vi "Main.vi"() -> ()   [LabVIEW 2013] (continued)
            n3896 = call <vilib>:"Application Directory.vi"() -> ("Application Directory"=w6305:path)
            n3897 = Build Path(base path=w6305, name or relative path="SRTRS.ini" ("ini Name")) -> (appended path=w6304:path)
            n3898 = call <vilib>:"Open Config Data.vi"("create file if necessary (T)"=FALSE, "configuration file path"=w6304) -> ("error out"=w6307:errorcluster, "refnum"=w6306:T59)  [unwired: 7 in, 1 out]
            n3899 = call-poly <vilib>:"Write Key.vi"("section"="Settings", "error in (no error)"=w6307, "value"="", "key"="Raw Data File", "refnum"=w6306) -> ("error out"=w6301:errorcluster, "found?"=w6300:bool, "refnum out"=w6299:T59)  [unwired: 4 in]
            n3900 = call <vilib>:"Close Config Data.vi"("error in (no error)"=w6301, "write file if changed (T)"=w6300, "refnum"=w6299) -> ("error out"=w6296:errorcluster)  [unwired: 7 in, 1 out]
            n3901 = local write "ini File Error"(w6296) -> ()
          }
        }
        n3902 = local read "Simulate cRIO"() -> (w6260:bool)
        n3903 = call "cRIO - Shared Variable RW.vi"("shared variable RT Library"=w6256, "Read/Write"=cRIO_RW_Enum."Write", "Error In"=w6258, "Simulate cRIO"=w6260, "DAQ Start"=FALSE, "cRIO Status"=w6247) -> ("Error Out"=w6261:errorcluster)  [unwired: 5 in, 8 out]
        n3904 = while {
          tunnel: w6261 -> [w6573]
          tunnel: w6260 -> [w6572]
          tunnel: w6247 -> [w6562]
          tunnel: w6256 -> [w6561]
          tunnel: [w6560] -> w6248
          i -> [w6567]
          stop <- w6569 stop-if-true
          # "Wait 5sec"
          # "Check for cRIO DAQ Stop"
          n3905 = Wait Until Next ms Multiple(millisecond multiple=u32 100) -> ()  [unwired: 1 out]
          n3906 = call "cRIO - Shared Variable RW.vi"("shared variable RT Library"=w6561, "Read/Write"=cRIO_RW_Enum."Read", "Error In"=w6573, "Simulate cRIO"=w6572, "cRIO Status"=w6562) -> ("Cycle Count"=w6570:i32, "DAQ Started"=w6563:bool, "Error Out"=w6560:errorcluster)  [unwired: 6 in, 6 out]
          n3907 = local write "cRIO Cycle Count"(w6570) -> ()
          n3908 = local write "cRIO DAQ Started"(w6563) -> ()
          n3909 = local write "cRIO Error"(w6560) -> ()
          n3910 = Not(x=w6563) -> (.not. x?=w6568:bool)
          n3911 = Greater Or Equal?(x=w6567, y=50) -> (x >= y?=w6565:bool)
          n3912 = Compound Arithmetic op=OR(w6565, w6568, w6560) -> (w6569:bool)
        }
        n3913 = global read "Global SRTRS.vi" "Logon"() -> (w6246:T21)
        n3914 = Unbundle By Name(w6246) -> ("PlantID"=w6245:string, "SystemID"=w6244:string)
        n3915 = Bundle("PlantID"=w6245, "SystemID"=w6244) -> (w6243:cluster{"PlantID":string, "SystemID":string})  [unwired: 1 in]
        n3916 = local read "DB - Transaction"() -> (w6251:bool)
        n3917 = call "Status - Update cRIO Status.vi"("Error In"=w6248, "[PlantId],[SystemId]"=w6243, "cRIO Status"=w6247) -> ("Error Out"=w6242:errorcluster)  [unwired: 8 in]
        n3918 = local write "System Status"(w6242) -> ()
        n3919 = case shown="No Error" w6249 {
          selector: w6249 -> [_ w6489]
          tunnel: w6250 -> [w6482 _]
          tunnel: [w6484 w6489] -> w6253
          frame No Error {
            # "Overwrite raw data from cRIO to Chart"
            n3920 = call "Chart - Load History.vi"("file path (dialog if empty)"=w6482) -> ("Error Out"=w6485:errorcluster, "History"=w6486:dynamicdata[])  [unwired: 5 in, 4 out]
            n3921 = property on="Chart" class="WFChart (strict)"(error in=w6485, "History Data"=w6486) -> (error out=w6484:errorcluster)  [unwired: 1 in, 1 out]
            n3922 = case shown="No Error" w6484 {
              tunnel: ["Raw Data File Load to Chart OK. " "Raw Data File Load to Chart failed. "] -> w6481
              frame No Error {
              }
              frame Error {
              }
            }
            n3923 = Path To String(path=w6482) -> (string=w6479:string)
            n3924 = Concatenate Strings("{END Recipe} ", w6481, " File: \"" ("string"), w6479, "\"" ("string")) -> (w6477:string)
            n3925 = call "Queue - EnQueue to MessageQ.vi"("<NoD> Don't Display to UI"=TRUE, "Message"=w6477) -> ()  [unwired: 9 in, 1 out]
          }
          frame Error {
          }
        }
        n3926 = case shown="True" w6251 {
          tunnel: w6250 -> [_ w6315]
          tunnel: w6249 -> [_ w6340]
          tunnel: w6241 -> [_ _]
          tunnel: w6240 -> [_ w6310]
          tunnel: [errorcluster {"status"=FALSE, "code"=0, "source"=""} ("error IO") w6314] -> w6239
          frame False {
          }
          frame True {
            w6327 = "0"  # IsActive
            w6344 = ""
            w6323 = "1"  # Process Complete
            w6360 = T62[] [enum."[EndRecordTemp]", enum."[EndRecordTime]", enum."[RecordedMinutes]", enum."[ProcessStatus]", enum."[OverallStatus]", enum."[Result]"] items=["[StartRecordTime]", "[StartRecordTemp]", "[MaxRecordedTemp]", "[MaxRecordedTempTime]", "[MinRecordedTemp]", "[MinRecordedTempTime]", "[EndRecordTemp]", "[EndRecordTime]", "[RecordedMinutes]", "[StartHoldTime]", "[StartHoldTemp]", "[HoldTimeMaxTemp]", "[HoldTimeMaxTempTime]", "[HoldTimeMinTemp]", "[HoldTimeMinTempTime]", "[EndHoldTime]", "[EndHoldTemp]", "[HoldDurationMinutes]", "[TempDiffDuringHold]", "[UnitOfTemperature]", "[PerformedBy]", "[PerformedOn]", "[IsTempWithinTol]", "[IsTimeWithinTol]", "[HoldTimePercentage]", "[ProcessStatus]", "[OverallStatus]", "[SequenceStatus]", "[Parameter1]", "[Parameter2]", "[Parameter3]", "[Parameter4]", "[Parameter5]", "[Parameter6]", "[Parameter7]", "[Parameter8]", "[Parameter9]", "[Parameter10]", "[Parameter11]", "[Parameter12]", "[Result]", "[RawDataFile]", "[RawDataFilePath]", "[RawDataFileName]", "[OutputSetId]", "[SavedBy]", "[SavedOn]", "[Inactive]"]  # [TransactionResult] Array
            # "Actuall should put whole thing in Error"
            # "Set in {Running Process} when it exited"
            n3927 = local read "[StartRecordTime]"() -> (w6355:string)
            n3928 = local read "Simulate cRIO"() -> (w6337:bool)
            n3929 = case shown="True" w6337 {
              tunnel: [w6372 w6376] -> w6336
              frame False {
                n3930 = Get Date/Time In Seconds() -> (seconds since 1Jan1904=w6372:timestamp)
              }
              frame True {
                # "Every count is 60sec"
                n3931 = local read "Process t0"() -> (w6377:timestamp)
                n3932 = local read "Samples/ch Count"() -> (w6373:i32)
                n3933 = Multiply(x=w6373, y=60) -> (x*y=w6374:i32)
                n3934 = Add(x=w6374, y=w6377) -> (x+y=w6376:timestamp)
              }
            }
            n3935 = call "Chart - Load History.vi"("file path (dialog if empty)"=w6315) -> ("t0 time stamp"=w6339:timestamp, "History"=w6338:dynamicdata[])  [unwired: 5 in, 4 out]
            n3936 = global read "Global SRTRS.vi" "Date Time Format"() -> (w6356:string)
            n3937 = call "String - Convert Str (YYYY-mm-dd HHcMMcSS) to TimeStamp.vi"("YYYY-mm-dd HH:MM:SS (String)"=w6355) -> ("time stamp"=w6335:timestamp)  [unwired: 9 in, 1 out]
            n3938 = Select(t="1", s=w6310, f="0") -> (s? t:f=w6318:string)
            n3939 = Select(t="1", s=w6310, f="0") -> (s? t:f=w6311:string)
            n3940 = Format Date/Time String(time format string (%c)=w6356, seconds (now)=w6336) -> (date/time string=w6330:string)  [unwired: 1 in]
            n3941 = local read "1st TC"() -> (w6358:dbl)
            n3942 = Subtract "Seconds"(x=w6336, y=w6335) -> (x-y=w6354:dbl)
            n3943 = Divide "Minutes"(x=w6354, y=60.0) -> (x/y=w6352:dbl)
            n3944 = Format Value(format string="%#_4", value (0)=w6358) -> (output string=w6357:string)  [unwired: 1 in]
            n3945 = Number To Decimal String(number=w6352) -> (decimal integer string=w6329:string)  [unwired: 1 in]
            n3946 = Build Array(w6357, w6330, w6329, w6323, w6318, w6311) -> (w6351:string[])
            n3947 = control-ref of="Process Completed"() -> (w6322:refnum<vi>)
            n3948 = control-ref of="Overall Status"() -> (w6317:refnum<vi>)
            n3949 = call "String - Boolean Ref Color.vi"("Bool Refnum"=w6322) -> ("Color (U32 String)"=w6321:string)  [unwired: 4 in]
            n3950 = call "String - Boolean Ref Color.vi"("Bool Refnum"=w6317) -> ("Color (U32 String)"=w6316:string)  [unwired: 4 in]
            n3951 = local read "Transaction No (Execute)"() -> (w6342:string)
            n3952 = local read "TransactionRunNo (Execute)"() -> (w6341:string)
            n3953 = Build Array(w6330, w6329, w6321, w6316, w6327) -> (w6328:string[])
            n3954 = Bundle("Transaction No (Execute)"=w6342, "TransactionRunNo (Execute)"=w6341) -> (w6334:T77)  [unwired: 1 in]
            n3955 = global read "Global SRTRS.vi" "Logon"() -> (w6346:T21)
            n3956 = call "DB - [Execute].[Transaction].vi"("DB.Schema.Table"="SRTRS.Execute.TransactionResult", "Transaction"=w6334, "DB - Execute Transaction"=DB_-_Execute_Transaction_Enum."UPDATE [TransactionResult]", "[TransactionResult] v02"=w6360, "<Values>"=w6351) -> ("SUMMARY"=w6347:errorcluster)  [unwired: 11 in, 3 out]
            n3957 = Unbundle By Name(w6346) -> ("PlantID"=w6349:string, "StationID"=w6348:string)
            n3958 = Build Array(w6349, w6348, w6344, w6344) -> (w6345:string[])
            n3959 = local read "Enable Central Monitoring"() -> (w6332:bool)
            n3960 = local read "DB - Active Process"() -> (w6333:bool)
            n3961 = call "DB - [Execute].[Transaction].vi"("DB.Schema.Table"="SRTRS.Execute.Active", "error in (no error)"=w6347, "DB - Execute Transaction"=DB_-_Execute_Transaction_Enum."INSERT/UPDATE [Execute].[Active]", "<Values>"=w6345) -> ("SUMMARY"=w6326:errorcluster)  [unwired: 12 in, 3 out]
            n3962 = And(x=w6332, y=w6333) -> (x .and. y?=w6331:bool)
            n3963 = case shown="True" w6331 {
              tunnel: w6328 -> [_ w6367]
              tunnel: [_ w6366] -> w6324
              frame False {
              }
              frame True {
                w6371 = T63[] [enum."[EndRecordTime]", enum."[RecordedMinutes]", enum."[ProcessColor]", enum."[OverallColor]", enum."[IsActive]"] items=["[IsActive]", "[TransactionNo]", "[TransactionRunNo]", "[SequenceStatus]", "[StartRecordTime]", "[EndRecordTime]", "[StartHoldTime]", "[EndHoldTime]", "[Message1]", "[Message2]", "[HoldTimeRemaining]", "[HoldTimePercentage]", "[HoldProgressColor]", "[OrderNumbers]", "[CurrentTemp]", "[UnitOfTemperature]", "[IsAppClientLive]", "[RawDataFile]", "[RecordedMinutes]", "[FurnaceControlStatus]", "[FurnaceControlColor]", "[ControllerStatus]", "[ControllerColor]", "[IsControllerOnline]", "[ProcessColor]", "[OverallColor]", "[LastUpdatedOn]", "[LastUpdatedCmsTime]", "[Inactive]"] ("[Execute].[ActiveProcess]\n2014-10-14 14:58")
                n3964 = global read "Global SRTRS.vi" "Logon"() -> (w6370:T21)
                n3965 = Unbundle By Name(w6370) -> ("PlantID"=w6369:string, "SystemID"=w6368:string)
                n3966 = Bundle("PlantID"=w6369, "SystemID"=w6368) -> (w6365:cluster{"PlantID":string, "SystemID":string})  [unwired: 1 in]
                n3967 = call "DB - [CMS].[Execute].[ActiveProcess].vi"("Application"="SRTRS", "[PlantId],[SystemId]"=w6365, "DB - CMS Execute ActiveProcess"=DB_-_CMS_Execute_Active_Process."UPDATE [Execute].[ActiveProcess]", "[Execute].[ActiveProcess]\n2014-10-14 14:58"=w6371, "<Data>"=w6367) -> ("SUMMARY"=w6366:errorcluster)  [unwired: 11 in, 3 out]
              }
            }
            n3968 = Merge Errors(w6324, w6326) -> (w6325:errorcluster)
            n3969 = case shown="No Error" w6340 {
              selector: w6340 -> [_ w6475]
              tunnel: w6338 -> [w6471 _]
              tunnel: w6339 -> [w6465 _]
              tunnel: w6325 -> [_ _]
              tunnel: w6334 -> [w6442 _]
              tunnel: w6315 -> [w6409 _]
              tunnel: [w6399 w6475] -> w6314
              frame No Error {
                w6440 = "%#_4" ("format string")
                w6423 = T62[] [enum."[MaxRecordedTemp]", enum."[MaxRecordedTempTime]", enum."[MinRecordedTemp]", enum."[MinRecordedTempTime]", enum."[TempDiffDuringHold]"] items=["[StartRecordTime]", "[StartRecordTemp]", "[MaxRecordedTemp]", "[MaxRecordedTempTime]", "[MinRecordedTemp]", "[MinRecordedTempTime]", "[EndRecordTemp]", "[EndRecordTime]", "[RecordedMinutes]", "[StartHoldTime]", "[StartHoldTemp]", "[HoldTimeMaxTemp]", "[HoldTimeMaxTempTime]", "[HoldTimeMinTemp]", "[HoldTimeMinTempTime]", "[EndHoldTime]", "[EndHoldTemp]", "[HoldDurationMinutes]", "[TempDiffDuringHold]", "[UnitOfTemperature]", "[PerformedBy]", "[PerformedOn]", "[IsTempWithinTol]", "[IsTimeWithinTol]", "[HoldTimePercentage]", "[ProcessStatus]", "[OverallStatus]", "[SequenceStatus]", "[Parameter1]", "[Parameter2]", "[Parameter3]", "[Parameter4]", "[Parameter5]", "[Parameter6]", "[Parameter7]", "[Parameter8]", "[Parameter9]", "[Parameter10]", "[Parameter11]", "[Parameter12]", "[Result]", "[RawDataFile]", "[RawDataFilePath]", "[RawDataFileName]", "[OutputSetId]", "[SavedBy]", "[SavedOn]", "[Inactive]"] ("[TransactionResult] v02")
                w6443 = "%#_4" ("format string")
                w6424 = T62[] [enum."[HoldTimeMaxTemp]", enum."[HoldTimeMaxTempTime]", enum."[HoldTimeMinTemp]", enum."[HoldTimeMinTempTime]", enum."[TempDiffDuringHold]"] items=["[StartRecordTime]", "[StartRecordTemp]", "[MaxRecordedTemp]", "[MaxRecordedTempTime]", "[MinRecordedTemp]", "[MinRecordedTempTime]", "[EndRecordTemp]", "[EndRecordTime]", "[RecordedMinutes]", "[StartHoldTime]", "[StartHoldTemp]", "[HoldTimeMaxTemp]", "[HoldTimeMaxTempTime]", "[HoldTimeMinTemp]", "[HoldTimeMinTempTime]", "[EndHoldTime]", "[EndHoldTemp]", "[HoldDurationMinutes]", "[TempDiffDuringHold]", "[UnitOfTemperature]", "[PerformedBy]", "[PerformedOn]", "[IsTempWithinTol]", "[IsTimeWithinTol]", "[HoldTimePercentage]", "[ProcessStatus]", "[OverallStatus]", "[SequenceStatus]", "[Parameter1]", "[Parameter2]", "[Parameter3]", "[Parameter4]", "[Parameter5]", "[Parameter6]", "[Parameter7]", "[Parameter8]", "[Parameter9]", "[Parameter10]", "[Parameter11]", "[Parameter12]", "[Result]", "[RawDataFile]", "[RawDataFilePath]", "[RawDataFileName]", "[OutputSetId]", "[SavedBy]", "[SavedOn]", "[Inactive]"] ("[TransactionResult] v02")
                w6468 = u16 1 items=["Samples", "Relative Time"] ("start/duration format")
                w6469 = 0  # TC0
                # "Use this Sequence with Recovery Flag to update \n- Variant Hold Time (Indicator)\n- Varaint Hold Temp (Indicator)\n- Overall Status (Indicator)\n- OverallStatus & Result (DB)\n(Already computed - ProcessStatus (DB))"
                # "Calculate Parameters from FTP-ed raw data from cRIO"
                n3970 = local read "Parameter Buffer"() -> (w6474:T15)
                n3971 = Unbundle By Name(w6474) -> ("Start Holding Time and Date"=w6473:string, "End Holding Time and Date"=w6472:string)  [unwired: 2 out]
                n3972 = Index Array(array=w6471, index=w6469) -> (element=w6470:dynamicdata)
                n3973 = call "Convert from Dynamic Data"("Dynamic Data Type"=w6470) -> ("Waveform"=w6441:waveform(dbl))  [unwired: 3 in]
                n3974 = call "String - Convert Str (YYYY-mm-dd HHcMMcSS) to TimeStamp.vi"("YYYY-mm-dd HH:MM:SS (String)"=w6473) -> ("time stamp"=w6467:timestamp)  [unwired: 9 in, 1 out]
                n3975 = call "String - Convert Str (YYYY-mm-dd HHcMMcSS) to TimeStamp.vi"("YYYY-mm-dd HH:MM:SS (String)"=w6472) -> ("time stamp"=w6466:timestamp)  [unwired: 9 in, 1 out]
                n3976 = Subtract(x=w6467, y=w6465) -> (x-y=w6463:dbl)
                n3977 = Subtract(x=w6466, y=w6465) -> (x-y=w6464:dbl)
                n3978 = Subtract(x=w6464, y=w6463) -> (x-y=w6397:dbl)
                n3979 = call-poly <vilib>:"Get Waveform Subset.vi"("start/duration format"=w6468, "duration"=w6397, "start samples/time"=w6463, "waveform in"=w6441) -> ("error out"=→"Chart":errorcluster, "waveform out"=w6461:waveform(dbl))  [unwired: 2 in, 2 out]
                n3980 = Divide "Hold Time (min)"(x=w6397, y=60.0) -> (x/y=w6395:dbl)
                n3981 = call "Statistics"("Signals"=w6461) -> ("Range"=w6455:dynamicdata, "Time of Minimum"=w6456:dynamicdata, "Minimum"=w6457:dynamicdata, "Time of Maximum"=w6458:dynamicdata, "Maximum"=w6459:dynamicdata, "error out"=w6417:errorcluster)  [unwired: 21 in]
                n3982 = call "Statistics2"("Signals"=w6441) -> ("Time of Minimum"=w6429:dynamicdata, "Minimum"=w6430:dynamicdata, "Time of Maximum"=w6431:dynamicdata, "Maximum"=w6432:dynamicdata, "error out"=w6416:errorcluster)  [unwired: 21 in, 1 out]
                n3983 = property on="Variant Allowed (Hold Temp)" class="DigNum (strict)"() -> ("Value"=w6380:dbl)  [unwired: 2 in, 2 out]
                n3984 = property on="Hold. Temp." class="Str"() -> ("Value"=w6390:string)  [unwired: 2 in, 2 out]
                n3985 = property on="Variant Allowed (Hold Time)" class="DigNum (strict)"() -> ("Value"=w6392:dbl)  [unwired: 2 in, 2 out]
                n3986 = property on="Hold. Time (hour:minute)" class="Str"() -> ("Value"=w6398:string)  [unwired: 2 in, 2 out]
                n3987 = Merge Errors(w6417, w6416) -> (→"Statistics":errorcluster)
                n3988 = call "String - (HH_colon_MM) to Minutes.vi"("Hold Time (HH:MM)"=w6398) -> ("minutes"=w6394:dbl)  [unwired: 10 in]
                n3989 = call "Convert from Dynamic Data7"("Dynamic Data Type"=w6432) -> ("Scalar"=w6428:dbl)  [unwired: 3 in]
                n3990 = call "Convert from Dynamic Data8"("Dynamic Data Type"=w6431) -> ("Scalar"=w6427:dbl)  [unwired: 3 in]
                n3991 = call "Convert from Dynamic Data9"("Dynamic Data Type"=w6430) -> ("Scalar"=w6426:dbl)  [unwired: 3 in]
                n3992 = call "Convert from Dynamic Data10"("Dynamic Data Type"=w6429) -> ("Scalar"=w6425:dbl)  [unwired: 3 in]
                n3993 = call "Convert from Dynamic Data2"("Dynamic Data Type"=w6459) -> ("Scalar"=w6389:dbl)  [unwired: 3 in]
                n3994 = call "Convert from Dynamic Data3"("Dynamic Data Type"=w6458) -> ("Scalar"=w6453:dbl)  [unwired: 3 in]
                n3995 = call "Convert from Dynamic Data4"("Dynamic Data Type"=w6457) -> ("Scalar"=w6388:dbl)  [unwired: 3 in]
                n3996 = call "Convert from Dynamic Data5"("Dynamic Data Type"=w6456) -> ("Scalar"=w6454:dbl)  [unwired: 3 in]
                n3997 = call "Convert from Dynamic Data6"("Dynamic Data Type"=w6455) -> ("Scalar"=w6445:dbl)  [unwired: 3 in]
                n3998 = global read "Global SRTRS.vi" "Date Time Format"() -> (w6433:string)
                n3999 = Fract/Exp String To Number(string=w6390) -> (number=w6387:dbl)  [unwired: 3 in, 1 out]
                n4000 = To Time Stamp(1:w6427) -> (0:w6434:timestamp)
                n4001 = To Time Stamp(1:w6453) -> (0:w6452:timestamp)
                n4002 = To Time Stamp(1:w6425) -> (0:w6436:timestamp)
                n4003 = To Time Stamp(1:w6454) -> (0:w6450:timestamp)
                n4004 = Subtract(x=w6395, y=w6394) -> (x-y=w6393:dbl)
                n4005 = Absolute Value(x=w6393) -> (abs(x)=w6391:dbl)
                "|Hold - Hold Time|" <- w6391
                n4006 = Format Value(format string=w6440, value (0)=w6428) -> (output string=w6438:string)  [unwired: 1 in]
                n4007 = Format Date/Time String(time format string (%c)=w6433, seconds (now)=w6434) -> (date/time string=w6435:string)  [unwired: 1 in]
                n4008 = Format Value(format string=w6443, value (0)=w6389) -> (output string=w6447:string)  [unwired: 1 in]
                n4009 = Format Date/Time String(time format string (%c)=w6433, seconds (now)=w6452) -> (date/time string=w6451:string)  [unwired: 1 in]
                n4010 = Format Value(format string=w6440, value (0)=w6426) -> (output string=w6439:string)  [unwired: 1 in]
                n4011 = Format Date/Time String(time format string (%c)=w6433, seconds (now)=w6436) -> (date/time string=w6437:string)  [unwired: 1 in]
                n4012 = Format Value(format string=w6443, value (0)=w6388) -> (output string=w6446:string)  [unwired: 1 in]
                n4013 = Format Date/Time String(time format string (%c)=w6433, seconds (now)=w6450) -> (date/time string=w6449:string)  [unwired: 1 in]
                n4014 = Format Value(format string=w6443, value (0)=w6445) -> (output string=w6444:string)  [unwired: 1 in]
                n4015 = Greater?(x=w6392, y=w6391) -> (0:→"Variant Allowed (Hold Time) (raw Data)":bool)
                n4016 = Build Array(w6438, w6435, w6439, w6437) -> (w6421:string[])
                n4017 = Build Array(w6447, w6451, w6446, w6449, w6444) -> (w6420:string[])
                n4018 = Build Array (concatenate)(w6420, w6421) -> (w6419:string[])
                "Calculate Parameters from raw Data" <- w6419
                n4019 = Subtract(x=w6389, y=w6387) -> (x-y=w6386:dbl)
                n4020 = Subtract(x=w6388, y=w6387) -> (x-y=w6385:dbl)
                n4021 = Absolute Value(x=w6386) -> (abs(x)=w6378:dbl)
                "|Max - Hold Temp|" <- w6378
                n4022 = Absolute Value(x=w6385) -> (abs(x)=w6379:dbl)
                "|Min - Hold Temp|" <- w6379
                n4023 = Greater?(x=w6380, y=w6378) -> (0:w6384:bool)
                n4024 = Greater?(x=w6380, y=w6379) -> (0:w6383:bool)
                n4025 = And(x=w6384, y=w6383) -> (x .and. y?=→"Variant Allowed (Hold Temp) (raw Data)":bool)
                n4026 = Build Array (concatenate)(w6424, w6423) -> (w6422:T62[])
                n4027 = call "DB - [Execute].[Transaction].vi"("DB.Schema.Table"="SRTRS.Execute.TransactionResult", "Transaction"=w6442, "DB - Execute Transaction"=DB_-_Execute_Transaction_Enum."UPDATE [TransactionResult]", "[TransactionResult] v02"=w6422, "<Values>"=w6419) -> ("Transaction"=w6402:T19, "SUMMARY"=w6404:errorcluster)  [unwired: 11 in, 2 out]
                n4028 = Open/Create/Replace File(file path (use dialog)=w6409, access (0:read/write)=enum16{"read/write", "read-only", "write-only"}."read-only") -> (refnum out=w6408:refnum<file>)  [unwired: 4 in, 2 out]
                n4029 = Set File Position(refnum=w6408, from (0:start)=enum16{"start", "end", "current"}."start") -> (refnum out=w6412:refnum<file>, error out=w6413:errorcluster)  [unwired: 2 in]
                n4030 = Read from Text File(file (use dialog)=w6412, count=-1, error in=w6413) -> (refnum out=w6405:refnum<file>, text=w6407:string, error out=w6406:errorcluster)  [unwired: 1 in, 1 out]
                n4031 = call "DB - [Execute].[Transaction].vi"("DB.Schema.Table"="SRTRS.Execute.TransactionResult", "String ([RawDataFile] Filestream)"=w6407, "Transaction"=w6402, "error in (no error)"=w6404, "DB - Execute Transaction"=DB_-_Execute_Transaction_Enum."UPDATE FILESTREAM") -> ("SUMMARY"=w6401:errorcluster)  [unwired: 11 in, 3 out]
                n4032 = local write "DB"(w6401) -> ()
                n4033 = Close File(refnum=w6405, error in=w6406) -> (error out=w6400:errorcluster)  [unwired: 1 out]
                n4034 = local write "Data File Error"(w6400) -> ()
                n4035 = Merge Errors(w6401, w6400) -> (w6399:errorcluster)
              }
              frame Error {
              }
            }
          }
        }
        n4036 = case shown="True" "Report.Create.Excel" {
          tunnel: w6259 -> [w6574 _]
          tunnel: [w6574 w6575] -> w6265
          tunnel: w6250 -> [_ w6576]
          tunnel: w6239 -> [_ _]
          frame False {
          }
          frame True {
            # "Create Excel Report"
            n4037 = flat-sequence {
              tunnel: w6576 -> [w6581]
              tunnel: [w6582] -> w6575
              frame #0 {
                # "Update Correct Transaction for Report\nSince this is immediately after a \nRUN, we will use the (Execute's) \nTranscation"
                # "This the raw data file from cRIO\n(unless cRIO is simulated)"
                n4038 = local write "Raw Data File (Report Tab)"(w6581) -> ()
                n4039 = local read "TransactionRunNo (Execute)"() -> (w6579:string)
                n4040 = local read "Transaction No (Execute)"() -> (w6580:string)
                n4041 = global read "Global SRTRS.vi" "Logon"() -> (→"Logon (Report Buffer)":T21)
                n4042 = Bundle("Transaction No (Execute)"=w6580, "TransactionRunNo (Execute)"=w6579) -> (→"Transaction (Report Buffer)":T77)  [unwired: 1 in]
              }
              frame #1 {
                # "Check if Dwell completed.\nIf not, most likely, user pressed\nStop Button"
                n4043 = local read "Parameter (End Dwell Time)"() -> (w6583:timestamp)
                n4044 = Equal?(x=w6583, y=timestamp(3471350400 s since 1904-01-01) ("Parameter (Start Dwell Time)")) -> (x = y?=w6585:bool)
                n4045 = case shown="False" w6585 {
                  tunnel: [TRUE ("T button?") w6600] -> w6586
                  frame False {
                    # "Hold Complete"
                  }
                  frame True {
                    # "Prompt for Report Generation if Hold NOT Complete"
                    n4046 = call "Msgbox - Message Handler.vi"("Short Description (When DB Not Available)"="Generate Report?", "Description (When DB Not Available)"="Hold process did not complete. Do you want to generate report?", "<.?....> Message Code"="<W 308>") -> ("MHandler Error"=w6601:errorcluster, "OK Out"=w6600:bool)  [unwired: 6 in, 1 out]
                    n4047 = local write "MHandler"(w6601) -> ()
                  }
                }
                n4048 = case shown="True" w6586 {
                  tunnel: [errorcluster {"status"=FALSE, "code"=0, "source"=""} ("error out") w6593] -> w6582
                  frame False {
                    n4049 = call "Queue - EnQueue to MessageQ.vi"("<NoD> Don't Display to UI"=TRUE, "Message"="{END Recipe} Generate Report. User click Cancel.") -> ()  [unwired: 9 in, 1 out]
                  }
                  frame True {
                    n4050 = local read "ReportList Cluster"() -> (w6592:T18)
                    n4051 = Bundle By Name(cluster=w6592, "[IsManual]"="0") -> (w6591:T18)
                    n4052 = local write "ReportList Cluster"(w6591) -> ()
                    n4053 = property on="Report Generate Toggle" class="Bool (strict)"() -> ("Value"=w6594:bool)  [unwired: 2 in, 2 out]
                    n4054 = Not(x=w6594) -> (.not. x?=w6595:bool)
                    n4055 = property on="Report Generate Toggle" class="Bool (strict)"("Val(Sgnl)"=w6595) -> (error out=w6593:errorcluster)  [unwired: 2 in, 1 out]
                  }
                }
              }
            }
          }
        }
        n4056 = Merge Errors(w6265) -> (w6264:errorcluster)
      }
      frame "ERROR Handling" {
        # "Segment.Type"
        # "Wait For RUN"
        # "State. Must always connect"
        # "Cycle Count. Not in use but leave it for future"
        # "Must Keep Sample/ch Count because the Error may have \ncome from RUNNING Process 1. We need to keep track\non the Count."
        # "Clear Error \nUnless MessageQ has an Error\nin which case the Program \nWill Quit"
        # "Clear Error, STOP Processes"
        n4057 = Unbundle By Name(w6606) -> ("code"=w6609:i32)
        n4058 = flat-sequence {
          frame #0 {
            # "STOP cRIO"
          }
        }
        n4059 = case shown="0, Default" w6609 {
          tunnel: [w6618 _] -> w6608
          tunnel: [_ w6673] -> w6607
          tunnel: [_ w6672] -> _
          tunnel: w6606 -> [w6613 _]
          tunnel: w6605 -> [w6620 _]
          frame 0, Default {
            # "Error From ET3500 and cRIO"
            # "State with Error"
            # "-1950679035"
            # "-1073807193"
            # "Normal Error, \nNot Serious, we clear error and go back to READY TO START"
            n4060 = local read "Show LabVIEW Error"() -> (w6621:bool)
            n4061 = local read "ET3500 Error"() -> (w6614:errorcluster)
            n4062 = local read "Data File Error"() -> (w6611:errorcluster)
            n4063 = local read "cRIO Error"() -> (w6615:errorcluster)
            n4064 = Merge Errors(w6615, w6614) -> (w6623:errorcluster)
            n4065 = disable-structure shown="Disabled" {
              frame Disabled {
                w6653 = T35 [enum."Page Enabled", enum."Page Enabled", enum."Page Enabled", enum."Page Enabled", enum."Page Enabled"] items=["Page Enabled", "Page Disabled", "Page Disabled & Grayed"]
                n4066 = property on="Tab Body" class="TabCtl (strict)"() -> ("Pages"=w6654:refnum<vi>[])  [unwired: 2 in, 2 out]
                n4067 = for {
                  tunnel: w6654 -> [w6656] mode=indexing
                  tunnel: w6653 -> [w6655] mode=indexing
                  n4068 = property class="Page"(reference=w6656, "PageEnb"=w6655) -> ()  [unwired: 1 in, 2 out]
                }
              }
              frame Enabled {
              }
            }
            n4069 = case shown="False" w6621 {
              tunnel: w6613 -> [_ w6652]
              frame False {
              }
              frame True {
                n4070 = call <vilib>:"Simple Error Handler.vi"("error in (no error)"=w6652) -> ()  [unwired: 4 in, 5 out]
              }
            }
            n4071 = case shown="Error" w6611 {
              selector: w6611 -> [_ w6627]
              tunnel: [_ w6624] -> w6610
              frame No Error {
              }
              frame Error {
                n4072 = Unbundle By Name(w6627) -> ("source"=w6625:string)  [unwired: 1 out]
                n4073 = Concatenate Strings(" File I/O  ERROR. \n" ("element"), w6625) -> (w6624:string)
              }
            }
            n4074 = case shown="Error" w6614 {
              selector: w6614 -> [_ w6671]
              tunnel: [_ w6668] -> w6617
              frame No Error {
              }
              frame Error {
                n4075 = Unbundle By Name(w6671) -> ("source"=w6669:string)  [unwired: 1 out]
                n4076 = control-ref of="ET3504 Status"() -> (w6666:refnum<vi>)
                n4077 = property class="Str"(reference=w6666, "Text.BG Color"=u32 16777216 ("ET3500 Transparent Color"), "Value"="Offline." ("ET3500 Program Status")) -> ()  [unwired: 1 in, 2 out]
                n4078 = Concatenate Strings(" ET3500 comm ERROR. \n" ("element"), w6669, "\n\n" ("string")) -> (w6668:string)
              }
            }
            n4079 = case shown="Error" w6615 {
              selector: w6615 -> [_ w6663]
              tunnel: [_ w6660] -> w6616
              frame No Error {
              }
              frame Error {
                n4080 = Unbundle By Name(w6663) -> ("source"=w6661:string)  [unwired: 1 out]
                n4081 = control-ref of="cRIO Status"() -> (w6658:refnum<vi>)
                n4082 = property class="Str"(reference=w6658, "Text.BG Color"=u32 16777216 ("ET3500 Transparent Color"), "Value"="Offline. " ("cRIO Status")) -> ()  [unwired: 1 in, 2 out]
                n4083 = Concatenate Strings(" cRIO comm ERROR. \n" ("element"), w6661) -> (w6660:string)
              }
            }
            n4084 = Unbundle By Name(w6613) -> ("source"=w6612:string)
            n4085 = Concatenate Strings(w6610, w6616, w6617) -> (w6622:string)
            n4086 = case shown="\"READY TO START\", Default" w6620 {
              tunnel: w6623 -> [w6632 w6642]
              tunnel: w6622 -> [w6631 w6644]
              tunnel: [errorcluster {"status"=FALSE, "code"=0, "source"=""} ("ET3500 Error") _] -> w6619
              tunnel: [Enum_-_SRTRS_State."READY TO START" ("Enum") Enum_-_SRTRS_State."RUNNING Process" ("Enum")] -> w6618
              tunnel: w6612 -> [_ w6643]
              frame "READY TO START", Default {
                # "Prompt Error"
                n4087 = case shown="Error" w6632 {
                  tunnel: w6631 -> [_ w6640]
                  frame No Error {
                  }
                  frame Error {
                    # "Error for cRIO and ET3500 ONLY\nFile I/O Error logged in their respective State."
                    n4088 = Concatenate Strings("{Error Handling}" ("string"), w6640) -> (w6634:string)
                    n4089 = local write "Tab Body"(Enum_-_Tabs."Setup" ("Tab Body")) -> ()
                    n4090 = call "Msgbox - Message Handler.vi"("Short Description (When DB Not Available)"="Communication Error", "Description (When DB Not Available)"="Cannot start process.", "<.?....> Message Code"="<E 301>") -> ("MHandler Error"=w6635:errorcluster)  [unwired: 6 in, 2 out]
                    n4091 = local write "MHandler"(w6635) -> ()
                    n4092 = call "Queue - EnQueue to MessageQ.vi"("<NoD> Don't Display to UI"=TRUE, "Message"=w6634) -> ()  [unwired: 9 in, 1 out]
                  }
                }
              }
              frame "RUNNING Process" {
                # "Continue to go back to the same STATE. \nOnly Status will update that there is an ERROR. User can still choose to STOP the Recipe or CLOSE the program."
                n4093 = case shown="Error" w6642 {
                  tunnel: w6644 -> [_ w6650]
                  tunnel: w6643 -> [_ w6648]
                  frame No Error {
                  }
                  frame Error {
                    # "For cRIO (and ET3500) Errors Only\nFile I/O error Logged at respective States"
                    n4094 = Concatenate Strings("{Error Handling} " ("element"), w6650, " {Error Source} " ("string"), w6648) -> (w6647:string)
                    n4095 = call "Queue - EnQueue to MessageQ.vi"("<NoD> Don't Display to UI"=TRUE, "Message"=w6647) -> ()  [unwired: 9 in, 1 out]
                  }
                }
              }
            }
            n4096 = flat-sequence {
              tunnel: w6619 -> [w6628]
              frame #0 {
                n4097 = local write "ET3500 Error"(w6628) -> ()
                n4098 = local write "Data File Error"(w6628) -> ()
                n4099 = local write "cRIO Error"(w6628) -> ()
              }
            }
          }
          frame -88888 {
            w6672 = " QUIT."  # Send to MessageQ
            w6673 = TRUE  # STOP While Loop
            # "No more next STATE"
            # "Serious Error,  QUIT Now"
          }
        }
        n4100 = flat-sequence {
          frame #0 {
            # "Clear RS232"
          }
        }
      }
      frame "QUIT" {
        # "IS THIS TRUE OR FALSE?"
        # "Nothing to STOP at ET3500 because the only iteraction is via cRIO COM port which\nis controlled by the HOST. Once the HOST stops, no more COM commands will be issued."
        # "Clear All Hardware States"
        n4101 = flat-sequence {
          frame #0 {
            n4102 = local read "cRIO DAQ Started"() -> (w6676:bool)
            n4103 = case shown="True" w6676 {
              frame False {
              }
              frame True {
                # "Stop DAQ Start"
                # "If cRIO DAQ Started already"
                n4104 = local read "cRIO shared variable RT Library"() -> (w6678:string)
                n4105 = local read "Simulate cRIO"() -> (w6681:bool)
                n4106 = control-ref of="cRIO Status"() -> (w6679:refnum<vi>)
                n4107 = call "cRIO - Shared Variable RW.vi"("shared variable RT Library"=w6678, "Read/Write"=cRIO_RW_Enum."Write", "Simulate cRIO"=w6681, "DAQ Start"=FALSE, "cRIO Status"=w6679) -> ("Error Out"=w6680:errorcluster)  [unwired: 6 in, 8 out]
                n4108 = local write "cRIO Error"(w6680) -> ()
              }
            }
            n4109 = local write "Quit Flag"(TRUE ("Quit Flag")) -> ()
          }
          frame #1 {
            n4110 = call "Queue - EnQueue to MessageQ.vi"("<NoD> Don't Display to UI"=TRUE, "Message"="QUIT" ("element")) -> ()  [unwired: 9 in, 1 out]
          }
        }
      }
    }
    "State Machine Error Out" <- w4367
    n4111 = Format Date/Time String(time format string (%c)="%b %d, %Y  %H:%M:%S") -> (date/time string=→"date/time string":string)  [unwired: 2 in]
    n4112 = case shown="No Error" w4367 {
      tunnel: w4371 -> [w4380 _]
      tunnel: [w4375 Enum_-_SRTRS_State."ERROR Handling" ("Enum")] -> w4366
      frame No Error {
        n4113 = local read "Recipe Stop Flag"() -> (w4374:bool)
        n4114 = local read "Quit Flag"() -> (w4373:bool)
        n4115 = Or(x=w4374, y=w4373) -> (x .or. y?=w4379:bool)
        n4116 = Select(t=Enum_-_SRTRS_State."END Recipe" ("Enum"), s=w4374, f=Enum_-_SRTRS_State."QUIT" ("Enum")) -> (s? t:f=w4376:T22)
        n4117 = Select(t=w4376, s=w4379, f=w4380) -> (s? t:f=w4375:T22)
      }
      frame Error {
      }
    }
    "StateMachine for Main Process" <- w4363
  }
  n4118 = disable-structure "Templates" shown="Disabled" {
    frame Disabled {
      w6689 = "{Save WPS Cancelled} ... must be entered." ("element")
      (unwired) path "C:/Temp1/SRTRS v2.0.0.50/VIs/Main_zh.xml" ("Read xml path")
      (unwired) path "C:/Temp1/SRTRS v2.0.0.50/VIs/Main.vi" ("VI path")
      n4119 = local read "Logon"() -> (w6698:T21)
      n4120 = Unbundle By Name(w6698) -> ()  [unwired: 1 out]
      n4121 = call "Queue - EnQueue to MessageQ.vi"("<NoD> Don't Display to UI"=TRUE, "Message"=w6689) -> ()  [unwired: 9 in, 1 out]
      n4122 = call "Msgbox UI.vi"("[ShortDescription] (Unicode)"=w6689, "[MessageType]"="E") -> ()  [unwired: 7 in, 3 out]
      n4123 = case shown="True" {
        selector: _ -> [_ _]
        tunnel: [w6710 w6714] -> _
        frame False {
          n4124 = Get Date/Time In Seconds() -> (seconds since 1Jan1904=w6710:timestamp)
        }
        frame True {
          # "Every count is 60sec"
          n4125 = local read "Process t0"() -> (w6715:timestamp)
          n4126 = local read "Samples/ch Count"() -> (w6711:i32)
          n4127 = Multiply(x=w6711, y=60) -> (x*y=w6712:i32)
          n4128 = Add(x=w6712, y=w6715) -> (x+y=w6714:timestamp)
        }
      }
      n4129 = call "Msgbox - Message Handler.vi"("Short Description (When DB Not Available)"="", "Description (When DB Not Available)"="", "<.?....> Message Code"="<     >") -> ()  [unwired: 6 in, 3 out]
      n4130 = call <vilib>:"Application Directory.vi"() -> ("Application Directory"=w6705:path)
      n4131 = Build Path(base path=w6705, name or relative path="SRTRS.ini" ("ini Name")) -> (appended path=w6706:path)
      n4132 = call <vilib>:"Open Config Data.vi"("create file if necessary (T)"=FALSE, "configuration file path"=w6706) -> ("error out"=w6703:errorcluster, "refnum"=w6704:T59)  [unwired: 7 in, 1 out]
      n4133 = call-poly <vilib>:"Write Key.vi"("section"="Settings", "error in (no error)"=w6703, "key"="Running Number", "refnum"=w6704) -> ("error out"=w6699:errorcluster, "refnum out"=w6700:T59)  [unwired: 5 in, 1 out]
      n4134 = call <vilib>:"Close Config Data.vi"("error in (no error)"=w6699, "refnum"=w6700) -> ("error out"=w6701:errorcluster)  [unwired: 8 in, 1 out]
      n4135 = local write "ini File Error"(w6701) -> ()
      n4136 = local read "Current VI's path"() -> (w6692:path)
      n4137 = control-ref of="MasterData\\Language"() -> (w6695:refnum<vi>)
      n4138 = call "String - Create Caption Paths.vi"("name or relative path"="Main.vi", "Current VI's path"=w6692, "Path in"=w6695) -> ("xml Path"=w6697:path, "VI Path"=w6693:path)  [unwired: 7 in]
      n4139 = call "Caption Main VI.vi"("Read/Write(T) XML"=FALSE, "Read xml path"=w6697, "VI path"=w6693) -> ()  [unwired: 8 in, 1 out]
    }
    frame Enabled {
    }
  }
  n4140 = Close File(refnum=w19, error in=w18) -> (error out=→"Event File Error":errorcluster)  [unwired: 1 out]
  n4141 = while {
    tunnel: w2 -> [_]
    stop <- w6718 stop-if-true
    n4142 = local read "Final Logoff Timer (s)"() -> (w6716:i32)
    n4143 = call "Elapsed Time2"("Time Target (s)"=w6716, "Reset"="Reset Log off Display Timer") -> ("Elapsed Time (s)"=w6720:dbl)  [unwired: 10 in, 7 out]
    n4144 = property on="Time To Log Off" class="Slide (strict)"("Scale.Maximum"=w6716, "Scale.Minimum"=0.0 ("Scale.Range:Minimum")) -> ()  [unwired: 2 in, 2 out]
    n4145 = Subtract(x=w6716, y=w6720) -> (x-y=→"Time To Log Off":dbl)
    n4146 = case shown="False" "Reset Log off Display Timer" {
      frame False {
      }
      frame True {
        n4147 = local write "Reset Log off Display Timer"(FALSE ("Reset")) -> ()
      }
    }
    n4148 = local read "Quit Flag"() -> (w6718:bool)
    n4149 = Wait Until Next ms Multiple(millisecond multiple=u32 200) -> ()  [unwired: 1 out]
  }
  n4150 = while {
    tunnel: w2 -> [_]
    stop <- w6729 stop-if-true
    # "At Least 10 sec"
    # "Event Structure For Log off Timer"
    n4151 = local read "Log Off Timer (s)"() -> (w6730:i32)
    n4152 = Max & Min(x=w6730, y=10) -> (max(x,y)=w6725:i32)  [unwired: 1 out]
    "Final Logoff Timer (s)" <- w6725
    n4153 = Multiply(x=w6725, y=1000) -> (x*y=w6724:i32)
    n4154 = event shown="[0] Timeout" {
      selector: _ -> [_ _ _]
      dyn-events: _ -> [_ _ _]
      timeout: w6724 -> [_ _ _]
      tunnel: [_ TRUE _] -> w6729
      tunnel: [_ _ TRUE] -> w6728
      event Timeout {
        n4155 = event-data() -> ()  [unwired: 1 in, 3 out]
        n4156 = local read "Tab Body"() -> (w6731:T1)
        n4157 = case shown="\"Execute\"" w6731 {
          frame "Logon", Default {
            # "Cannot be Logon Screen"
          }
          frame "Execute" {
            w6737 = cluster{"Color Box":u32, "Color Box 2":u32}[] [{"Color Box"=16383786, "Color Box 2"=16383786}, {"Color Box"=6618880, "Color Box 2"=6618880}, {"Color Box"=4934475, "Color Box 2"=4934475}, {"Color Box"=6618880, "Color Box 2"=6618880}]  # Start Recipe
            n4158 = property on="Process Completed" class="Bool (strict)"() -> ("Colors [4]"=w6738:cluster{u32, u32}[], "Value"=w6736:bool)  [unwired: 2 in, 2 out]
            n4159 = Equal?(x=w6738, y=w6737) -> (x = y?=w6734:bool)
            n4160 = Equal?(x=w6736, y=FALSE) -> (x = y?=w6733:bool)
            n4161 = And(x=w6734, y=w6733) -> (x .and. y?=w6732:bool)
            n4162 = case shown="True" w6732 {
              frame False {
              }
              frame True {
                n4163 = local read "Current VI's path"() -> (w6741:path)
                n4164 = local read "User"() -> (w6739:string)
                n4165 = call "DB UI - Logon (Popup).vi"("User"=w6739, "Application"="SRTRS", "Main.vi VI's Path"=w6741) -> ()  [unwired: 9 in]
              }
            }
          }
        }
      }
      event "Stop Log off Event Structure": Value Change {
        n4166 = event-data() -> ()  [unwired: 1 in, 6 out]
      }
      event Mouse Move; Key Down {
        n4167 = event-data() -> ()  [unwired: 1 in, 3 out]
      }
    }
    n4168 = local write "Reset Log off Display Timer"(w6728) -> ()
  }
  n4169 = disable-structure "Templates" shown="Disabled" {
    frame Disabled {
      n4170 = case shown="Error" {
        selector: _ -> [_ _]
        tunnel: _ -> [w6758 _]
        tunnel: [w6754 w6761] -> _
        tunnel: "[Save WPS]" ("string") -> [w6752 w6760]
        frame No Error {
          w6756 = "\"" ("string")
          # "File Save OK"
          n4171 = Path To String(path=w6758) -> (string=w6757:string)
          n4172 = Concatenate Strings(w6752, " OK." ("string"), "\n") -> (w6751:string)
          n4173 = Concatenate Strings(w6751, w6756, w6757, w6756, " saved. " ("string")) -> (w6754:string)
        }
        frame Error {
          # "File Save Not OK"
          n4174 = Concatenate Strings(w6760, " Cancelled.", "\n") -> (w6761:string)
        }
      }
      n4175 = local read "CellBG Unused Cells"() -> (w6744:u32)
      n4176 = local read "CellBG New Cells"() -> (w6745:u32)
      n4177 = Concatenate Strings("Confirm Delete " ("string")) -> (w6748:string)  [unwired: 1 in]
      n4178 = Two Button Dialog(message=w6748) -> ()  [unwired: 2 in, 1 out]
      n4179 = call "MCListbox Refresh.vi"("Which Cells"=T46."Exisiting and Blank Cells", "color of New Cells"=w6745, "color of Blank cells"=w6744) -> ()  [unwired: 7 in, 2 out]
    }
    frame Enabled {
    }
  }
  n4180 = Merge Errors(w5, w4) -> (w3:errorcluster)
  n4181 = flat-sequence {
    tunnel: [w6764] -> w5
    tunnel: w7 -> [_]
    frame #0 {
      # "If the Main Loop was not stopped due to user clicking on QUIT button, we need to Create Quit Event to STOP Edit Recipe Event Loop."
      n4182 = property on="Close" class="Bool (strict)"("Val(Sgnl)"=TRUE ("Value (Signaling)")) -> (error out=w6764:errorcluster)  [unwired: 2 in, 1 out]
    }
  }
  n4183 = flat-sequence {
    tunnel: w3 -> [w6777]
    tunnel: [w6777] -> w8
    frame #0 {
      # "Here we want to FIRE Event in subPanel"
      # "Stop and Close SubPanels"
      n4184 = local read "Admin Equipment UI"() -> (w6769:refnum<vi>)
      n4185 = local read "Admin User UI"() -> (w6775:refnum<vi>)
      n4186 = control-ref of="Config UI"() -> (w6774:refnum<vi>)
      n4187 = control-ref of="Equipment UI"() -> (w6770:refnum<vi>)
      n4188 = control-ref of="Logon UI"() -> (w6768:refnum<vi>)
      n4189 = control-ref of="Output Details UI"() -> (w6765:refnum<vi>)
      n4190 = control-ref of="Admin User UI"() -> (w6773:refnum<vi>)
      n4191 = local read "Config UI"() -> (w6776:refnum<vi>)
      n4192 = local read "Layout UI"() -> (w6766:refnum<vi>)
      n4193 = local read "Logon UI"() -> (w6767:refnum<vi>)
      n4194 = Build Array(w6774, w6773, w6770, w6768, w6765) -> (w6771:refnum<vi>[])
      n4195 = Build Array(w6776, w6775, w6769, w6767, w6766) -> (w6772:refnum<vi>[])
      n4196 = for {
        tunnel: [w6782] -> w6779 mode=indexing
        tunnel: w6771 -> [w6781] mode=indexing
        tunnel: w6772 -> [w6780] mode=indexing
        n4197 = property class="VI"(reference=w6780) -> (reference out=w6785:refnum<vi>, error out=w6784:errorcluster, "Panel"=w6787:refnum<vi>)  [unwired: 1 in]
        n4198 = property class="Pnl"(reference=w6787, error in=w6784) -> (error out=w6783:errorcluster, "Controls[]"=w6786:refnum<vi>[])  [unwired: 1 out]
        n4199 = invoke on="Invoke Node" class="SubPnl" method="Remove VI"(reference=w6781, error in=w6783) -> (error out=w6789:errorcluster)  [unwired: 1 in, 2 out]
        n4200 = control-ref of="Stop"() -> (w6788:refnum<vi>)
        n4201 = call "subPanel - UI Fires Event.vi"("Val(Sgnl)"=TRUE, "Error In"=w6789, "Pnl Controls[]"=w6786, "CtlRef"=w6788) -> ("Error Out"=w6790:errorcluster)  [unwired: 5 in, 2 out]
        n4202 = Close Reference(reference=w6785, error in (no error)=w6790) -> (error out=w6782:errorcluster)
      }
      n4203 = Merge Errors(w6779, w6777) -> (w6778:errorcluster)
      n4204 = local write "UI Event"(w6778) -> ()
    }
  }
  n4205 = flat-sequence {
    tunnel: w11 -> [_]
    tunnel: w6 -> [_]
    frame #0 {
      n4206 = local read "Application:Name"() -> (w6797:string)
      n4207 = To Upper Case(1:w6797) -> (0:w6796:string)
      n4208 = To Upper Case(1:"LabVIEW.exe" ("regular expression")) -> (0:w6794:string)
      n4209 = Match Pattern(string=w6796, regular expression=w6794) -> (offset past match=w6793:i32)  [unwired: 1 in, 3 out]
      n4210 = Greater Or Equal To 0?(x=w6793) -> (x >= 0?=w6792:bool)
      n4211 = case shown="False" w6792 {
        frame False {
          # "Executable"
          n4212 = control-ref of="This VI"() -> (w6798:refnum<vi>)
          n4213 = invoke class="VI" method="FP.Close"(reference=w6798) -> ()  [unwired: 2 in, 3 out]
        }
        frame True {
          # "Show Debug TAB"
          # "LabVIEW Development"
          n4214 = property on="Tab Body" class="TabCtl (strict)"() -> ("Pages"=w6799:refnum<vi>[])  [unwired: 2 in, 2 out]
          n4215 = for {
            tunnel: w6799 -> [w6804] mode=indexing
            n4216 = property class="Page"(reference=w6804) -> (reference out=w6800:refnum<vi>, "PageLabel"=w6803:string)  [unwired: 1 in, 1 out]
            n4217 = Equal?(x=w6803, y="Debug") -> (x = y?=w6801:bool)
            n4218 = case shown="True" w6801 {
              tunnel: w6800 -> [_ w6806]
              frame False {
              }
              frame True {
                n4219 = property class="Page"(reference=w6806, "PageVis"=TRUE) -> ()  [unwired: 1 in, 2 out]
              }
            }
          }
        }
      }
    }
  }
  n4220 = flat-sequence {
    tunnel: w20 -> [w6810]
    tunnel: [w6808] -> w11
    tunnel: w8 -> [_]
    frame #0 {
      # "MessageQ is the last to release\nMSGBox to release also"
      n4221 = call "Msgbox - Release Q.vi"() -> ("Error Out"=w6807:errorcluster)  [unwired: 11 in]
      n4222 = local write "Close"(FALSE ("Quit")) -> ()
      n4223 = Release Queue "MessageQ"(queue=w6810) -> (error out=w6808:errorcluster)  [unwired: 2 in, 2 out]
      n4224 = local write "Msgbox"(w6807) -> ()
    }
  }
